vi "均匀DAC.vi"(8 "量化阶 V":dbl=0.02, 11 "数字编码":dbl[](array[numeric])) -> (2 "x+y":dbl)   [LabVIEW 2020]
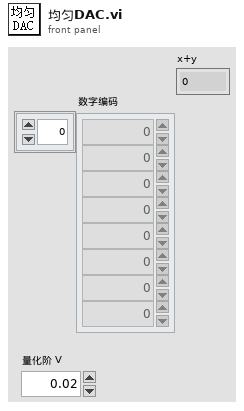
[diagram p1: front panel]
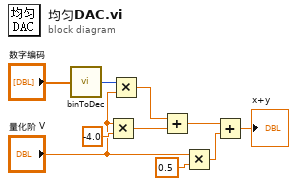
[diagram p0: block diagram]
diagram:
  n1 = call "binToDec.vi"("Array 2"="数字编码") -> ("output"=w9:i32)
  n2 = Multiply(x="量化阶 V", y=-4.0) -> (x*y=w6:dbl)
  n3 = Multiply(x=w9, y="量化阶 V") -> (x*y=w7:dbl)
  n4 = Add(x=w7, y=w6) -> (x+y=w5:dbl)
  n5 = Multiply(x="量化阶 V", y=0.5) -> (x*y=w2:dbl)
  n6 = Add(x=w5, y=w2) -> (x+y=→"x+y":dbl)
